vi "5_VisualAD_HyperParam_Search.vi"() -> ()   [LabVIEW 2020]
uses:
  <vilib>/Ngene/DeepLTK Anomaly Detection Addon/Toolkit/API/Controls/NNPC_Coreset_Params.ctl
  <vilib>/Ngene/DeepLTK Anomaly Detection Addon/Toolkit/API/Controls/NNPC_Setup.ctl
  <vilib>/Ngene/Deep Learning Toolkit/Toolkit/NN_Data/API/NN_Dims(C,H,W).ctl
  <vilib>/Ngene/Deep Learning Toolkit/Toolkit/NN_Network/Controls/NN_Device.ctl
  <vilib>/Ngene/DeepLTK Anomaly Detection Addon/Toolkit/API/Controls/Feature_Scorer_Params.ctl
  <vilib>/Ngene/DeepLTK Anomaly Detection Addon/Toolkit/API/Controls/Gaussian_Blur.ctl
  <vilib>/Ngene/DeepLTK Anomaly Detection Addon/Toolkit/API/Controls/Evaluation_Metrics.ctl
  <vilib>/Ngene/DeepLTK Anomaly Detection Addon/Toolkit/API/Controls/Eval_Results.ctl
  <vilib>/Ngene/DeepLTK Anomaly Detection Addon/Toolkit/API/Controls/MinMax.ctl
  <vilib>/Ngene/DeepLTK Anomaly Detection Addon/Toolkit/API/Controls/NNPC_Random_Projection_CFG.ctl
  <vilib>/Ngene/DeepLTK Anomaly Detection Addon/Toolkit/API/Controls/Dim_Reduction_Method.ctl
  <vilib>/Ngene/DeepLTK Anomaly Detection Addon/Toolkit/API/Controls/NNFE_CFG.ctl
  <vilib>/Ngene/DeepLTK Anomaly Detection Addon/Toolkit/API/Controls/Layer_Selector.ctl
  <vilib>/Ngene/DeepLTK Anomaly Detection Addon/Toolkit/API/Controls/Feature_Layer_Selector.ctl
  <vilib>/Ngene/DeepLTK Anomaly Detection Addon/Toolkit/API/Controls/Interpolation_Selector.ctl
  subVIs/Dataset_Reader/Controls/Read_Options.ctl
  <vilib>/Ngene/DeepLTK Anomaly Detection Addon/Toolkit/API/Controls/NNPC_PreProcessing_Options.ctl
  <vilib>/Ngene/DeepLTK Anomaly Detection Addon/Toolkit/API/Controls/NNPC_DS_Stats.ctl
  <vilib>/Ngene/DeepLTK Anomaly Detection Addon/Toolkit/API/Controls/Image_Stats_RGB.ctl
  subVIs/HyperParam_Search/Controls/Model_Info_and_Report.ctl
  subVIs/HyperParam_Search/Controls/Feature_Layers_CFG.ctl
  <vilib>/Ngene/DeepLTK Anomaly Detection Addon/Toolkit/API/Controls/Eval_Config.ctl
  <vilib>/Ngene/DeepLTK Anomaly Detection Addon/Toolkit/API/NNPC_Generate_Embedding/NNPC_Generate_Embedding(Dataset).vi
  <vilib>/Ngene/DeepLTK Anomaly Detection Addon/Toolkit/API/NNPC_Predict/NNPC_Predict(Dataset).vi
  <vilib>/Ngene/Deep Learning Toolkit/Toolkit/NN_Data/subVIs/Dataset_Destroy/NN_Dataset_Destroy(In3D_Out3D).vi
  <vilib>/Ngene/DeepLTK Anomaly Detection Addon/Toolkit/DeepLTK_Anomaly_Detection_Addon.lvlib
  <vilib>/Ngene/Deep Learning Toolkit/Toolkit/Deep_Learning_Toolkit_by_Ngene.lvlib
panel:
  in  "Tab Control":enum32{"Setup", "Results"}(tab)
  in  "Min_Layers_In_Group":u16=1
  in  "Dataset_Path(Train/Test/GT)":path=path "D:/Ngene/GitHub/deepltk_examples/3_Image_Processing/36_Anomaly_Detection/Dataset/Playing_Cards_3ofHearts"
  in  "Destination_Path":path=path "D:/working"
  in  "Coreset_Size":i32[](array[numeric])=[1000, 2000, 5000, 10000]
  in  "Proj._Dim.":i32[](array[numeric])=[128, 256, 512]
  in  "Coreset_Params":T1={"CoreSet_Size"=1.0, "Start_idx"=3}
  in  "NNPC_Setup":T2={"Input_Dims"={"C"=3, "H"=224, "W"=224}, "mBatch"=1, "Device"=enum."GPU", "GPU Id"=0}
  in  "Feature_Scorer_Params":T5={"Nearest_Neighbors"=1, "Calculate Anomaly Map"=FALSE, "Gaussian_Blur"={"Kernel_Size"=33, "Sigma"=4.0}}
  in  "Dim Reduction":T7={"Method"=enum."Rnd_Proj", "Target_Dim"=-1, "Seed"=42}
  in  "NNFE_CFG":T9={"Name"="", "Layer_Selection_By"=enum."Stride", "Feature_Layers"={"[LayerID, PatchSize]"=[{"Layer_ID"=8, "Patch_Size"=3}, {"Layer_ID"=16, "Patch_Size"=3}]}, "Interpolation_Type"=enum."Bi-Linear"}
  in  "NNFE_Folder_Paths":path[](array[path])=[path "D:/Ngene/GitHub/deepltk_examples/3_Image_Processing/36_Anomaly_Detection/NNFE/WRN_50_2_2_L3"]
  in  "Patch Sizes":i32[](array[numeric])=[1, 3, 5]
  in  "Layer ID":i32[](array[numeric])=[8, 16]
  out "Generated_Feature_Layers":T11[](array[typedef])=[{"[LayerID, PatchSize]"=[{"Layer_ID"=16, "Patch_Size"=1}]}, {"[LayerID, PatchSize]"=[{"Layer_ID"=16, "Patch_Size"=3}]}, {"[LayerID, PatchSize]"=[{"Layer_ID"=16, "Patch_Size"=5}]}, {"[LayerID, PatchSize]"=[{"Layer_ID"=8, "Patch_Size"=1}]}, {"[LayerID, PatchSize]"=[{"Layer_ID"=8, "Patch_Size"=1}, {"Layer_ID"=16, "Patch_Size"=1}]}, {"[LayerID, PatchSize]"=[{"Layer_ID"=8, "Patch_Size"=1}, {"Layer_ID"=16, "Patch_Size"=3}]}, {"[LayerID, PatchSize]"=[{"Layer_ID"=8, "Patch_Size"=1}, {"Layer_ID"=16, "Patch_Size"=5}]}, {"[LayerID, PatchSize]"=[{"Layer_ID"=8, "Patch_Size"=3}]}, {"[LayerID, PatchSize]"=[{"Layer_ID"=8, "Patch_Size"=3}, {"Layer_ID"=16, "Patch_Size"=1}]}, {"[LayerID, PatchSize]"=[{"Layer_ID"=8, "Patch_Size"=3}, {"Layer_ID"=16, "Patch_Size"=3}]}, {"[LayerID, PatchSize]"=[{"Layer_ID"=8, "Patch_Size"=3}, {"Layer_ID"=16, "Patch_Size"=5}]}, {"[LayerID, PatchSize]"=[{"Layer_ID"=8, "Patch_Size"=5}]}, {"[LayerID, PatchSize]"=[{"Layer_ID"=8, "Patch_Size"=5}, {"Layer_ID"=16, "Patch_Size"=1}]}, {"[LayerID, PatchSize]"=[{"Layer_ID"=8, "Patch_Size"=5}, {"Layer_ID"=16, "Patch_Size"=3}]}, {"[LayerID, PatchSize]"=[{"Layer_ID"=8, "Patch_Size"=5}, {"Layer_ID"=16, "Patch_Size"=5}]}]
  in  "Max_Layers_In_Group":u16=2
  out "error out":errorcluster
  in  "Img Res. H":i32[](array[numeric])=[224, 256]
  in  "Img Res. W":i32[](array[numeric])=[224, 256]
  in  "Single DS?":bool=TRUE
  out "Img._W":i32=224
  out "Elapsed Time":dbl=122.46820600000501 format="%<%H:%M:%S>t"
  out "Max_Dist":sgl[](graph)
  out "Tot Itr of one DS":i32=360
  out "Current Iter":i32=72
  out "Coreset Size":i32=4
  out "Proj. Dim.":i32=3
  out "Img Res.":i32=2
  out "Feature_Layers":i32=15
  out "Elapsed Time":dbl=122.46820600000501
  out "Evaluation_Metrics(Image)":T13={"Scores(Good)"={"X Values"=[48.00461868286133, 48.32544052124023, 48.64626235961914, 48.96708419799805, 49.28790603637695, 49.60872787475586, 49.92954971313476, 50.25037155151367, 50.57119338989258, 50.89201522827148, 51.212837066650394, 51.5336589050293, 51.8544807434082, 52.17530258178711, 52.49612442016601, 52.816946258544924, 53.13776809692383, 53.45858993530273, 53.779411773681645, 54.10023361206055, 54.421055450439454, 54.74187728881836, 55.06269912719726, 55.383520965576174, 55.70434280395508, 56.02516464233398, 56.34598648071289, 56.6668083190918, 56.987630157470704, 57.30845199584961, 57.62927383422851, 57.950095672607425, 58.27091751098633, 58.591739349365234, 58.91256118774414, 59.23338302612305, 59.554204864501955, 59.87502670288086, 60.195848541259764, 60.516670379638676, 60.83749221801758, 61.158314056396485, 61.47913589477539, 61.7999577331543, 62.120779571533205, 62.44160140991211, 62.762423248291014, 63.083245086669926, 63.40406692504883, 63.724888763427735, 64.04571060180663, 64.36653244018555, 64.68735427856446, 65.00817611694336, 65.32899795532227, 65.64981979370117, 65.97064163208009, 66.29146347045898, 66.6122853088379, 66.93310714721679, 67.2539289855957, 67.57475082397461, 67.89557266235352, 68.21639450073243, 68.53721633911132, 68.85803817749024, 69.17886001586913, 69.49968185424805, 69.82050369262694, 70.14132553100586, 70.46214736938477, 70.78296920776367, 71.10379104614259, 71.42461288452148, 71.7454347229004, 72.06625656127929, 72.38707839965821, 72.70790023803711, 73.02872207641602, 73.34954391479492, 73.67036575317383, 73.99118759155274, 74.31200942993163, 74.63283126831055, 74.95365310668944, 75.27447494506836, 75.59529678344727, 75.91611862182617, 76.23694046020509, 76.55776229858398, 76.8785841369629, 77.19940597534179, 77.52022781372071, 77.84104965209961, 78.16187149047852, 78.48269332885742, 78.80351516723633, 79.12433700561525, 79.44515884399414, 79.76598068237305], "Histogram: h(x)"=[1, 0, 0, 0, 0, 0, 1, 0, 0, 0, 1, 0, 1, 0, 1, 0, 2, 2, 0, 0, 1, 2, 1, 0, 0, 0, 1, 1, 0, 1, 0, 0, 0, 0, 1, 0, 0, 0, 1, 0, 0, 1, 0, 0, 1, 0, 0, 0, 0, 0, 0, 0, 0, 0, 0, 1, 0, 0, 0, 0, 0, 0, 0, 0, 0, 0, 0, 1, 0, 1, 1, 0, 0, 0, 0, 0, 0, 0, 0, 0, 0, 1, 0, 0, 0, 0, 0, 0, 0, 0, 0, 0, 0, 0, 0, 0, 0, 0, 0, 0]}, "Scores(Bad)"={"X Values"=[48.00461868286133, 48.32544052124023, 48.64626235961914, 48.96708419799805, 49.28790603637695, 49.60872787475586, 49.92954971313476, 50.25037155151367, 50.57119338989258, 50.89201522827148, 51.212837066650394, 51.5336589050293, 51.8544807434082, 52.17530258178711, 52.49612442016601, 52.816946258544924, 53.13776809692383, 53.45858993530273, 53.779411773681645, 54.10023361206055, 54.421055450439454, 54.74187728881836, 55.06269912719726, 55.383520965576174, 55.70434280395508, 56.02516464233398, 56.34598648071289, 56.6668083190918, 56.987630157470704, 57.30845199584961, 57.62927383422851, 57.950095672607425, 58.27091751098633, 58.591739349365234, 58.91256118774414, 59.23338302612305, 59.554204864501955, 59.87502670288086, 60.195848541259764, 60.516670379638676, 60.83749221801758, 61.158314056396485, 61.47913589477539, 61.7999577331543, 62.120779571533205, 62.44160140991211, 62.762423248291014, 63.083245086669926, 63.40406692504883, 63.724888763427735, 64.04571060180663, 64.36653244018555, 64.68735427856446, 65.00817611694336, 65.32899795532227, 65.64981979370117, 65.97064163208009, 66.29146347045898, 66.6122853088379, 66.93310714721679, 67.2539289855957, 67.57475082397461, 67.89557266235352, 68.21639450073243, 68.53721633911132, 68.85803817749024, 69.17886001586913, 69.49968185424805, 69.82050369262694, 70.14132553100586, 70.46214736938477, 70.78296920776367, 71.10379104614259, 71.42461288452148, 71.7454347229004, 72.06625656127929, 72.38707839965821, 72.70790023803711, 73.02872207641602, 73.34954391479492, 73.67036575317383, 73.99118759155274, 74.31200942993163, 74.63283126831055, 74.95365310668944, 75.27447494506836, 75.59529678344727, 75.91611862182617, 76.23694046020509, 76.55776229858398, 76.8785841369629, 77.19940597534179, 77.52022781372071, 77.84104965209961, 78.16187149047852, 78.48269332885742, 78.80351516723633, 79.12433700561525, 79.44515884399414, 79.76598068237305], "Histogram: h(x)"=[0, 0, 0, 0, 0, 0, 0, 0, 0, 0, 0, 0, 0, 0, 0, 0, 0, 0, 0, 0, 0, 0, 0, 0, 0, 0, 0, 0, 0, 0, 0, 0, 0, 0, 0, 0, 0, 0, 0, 0, 0, 0, 0, 0, 0, 0, 0, 0, 0, 0, 0, 0, 0, 0, 0, 0, 0, 0, 1, 0, 0, 0, 0, 0, 0, 1, 0, 0, 1, 3, 0, 1, 0, 1, 2, 0, 1, 0, 3, 2, 1, 1, 0, 2, 0, 1, 1, 0, 0, 1, 0, 0, 0, 0, 1, 0, 0, 0, 0, 1]}, "Eval Stats"={"Scores(Good)"={"Min"=47.844208, "Max"=73.85858}, "Scores(Bad)"={"Min"=66.62182, "Max"=79.92639}, "# of Samples(Good)"=25, "# of Samples(Bad)"=25, "AUROC"=0.9544, "F1_Max"=0.92592597, "Thrshld(F1_Max)"=65.82822, "Prec.(F1_Max)"=0.86206895, "Recall(F1_Max)"=1.0, "FPR(F1_Max)"=0.16, "FNR(F1_Max)"=0.0}} {"Eval Stats"."Recall(F1_Max)" format="%#.5f"; "Eval Stats"."FPR(F1_Max)" format="%#.5f"; "Eval Stats"."FNR(F1_Max)" format="%#.5f"; "Eval Stats"."Prec.(F1_Max)" format="%#.5f"; "Eval Stats"."F1_Max" format="%#.5f"; "Eval Stats"."AUROC" format="%#.5f"; "Eval Stats"."Scores(Bad)"."Min" format="%#_5g"; "Eval Stats"."Scores(Good)"."Min" format="%#_5g"; "Eval Stats"."Thrshld(F1_Max)" format="%#_5f"}
  out "Evaluation_Metrics(Pixel)":T13 {"Eval Stats"."Recall(F1_Max)" format="%#.5f"; "Eval Stats"."FPR(F1_Max)" format="%#.5f"; "Eval Stats"."FNR(F1_Max)" format="%#.5f"; "Eval Stats"."Prec.(F1_Max)" format="%#.5f"; "Eval Stats"."F1_Max" format="%#.5f"; "Eval Stats"."AUROC" format="%#.5f"; "Eval Stats"."Scores(Bad)"."Min" format="%#_5g"; "Eval Stats"."Scores(Good)"."Min" format="%#_5g"; "Eval Stats"."Thrshld(F1_Max)" format="%#_5f"}
  out "Coreset Size":i32
  out "Coreset Size":i32=10000
  out "Proj. Dim.":i32=128
  out "Img._H":i32=224
  out "Proj. Dim.":i32
  out "Img Res.":i32
  out "dT_Eval":dbl=0.0058932999963872135 format="%#_4p"
  out "dT_Inference":dbl=0.00638807999988785 format="%#_4p"
  out "dT_Coreset":dbl=3.193082099998719 format="%#_4p"
  out "dT_Embed":dbl=0.3958723999967333 format="%#_3p"
  out "dT_Init":dbl=1.9861645999917528 format="%#_3p"
  out "dT_DS_Read(Test)":dbl=0.14525060000596568 format="%#_3p"
  out "dT_DS_Read(Train)":dbl=0.18623009999282658 format="%#_3p"
  out "DS Size(Test)":i32=50
  out "DS Size(Train)":i32=50
  out "Feature_Layers":i32=6
  out "dT_DS_Read(Train)":dbl=0.18623009999282658 format="%#.0f"
  out "dT_DS_Read(Test)":dbl=0.14525060000596568 format="%#.0f"
  out "dT_Init":dbl=34.90064259998326 format="%#.0f"
  out "dT_Predict":dbl=21.941430500039132 format="%#.0f"
  out "dT_Coreset":dbl=53.35089359995618 format="%#.0f"
  out "dT_Embed":dbl=7.164398699984304 format="%#.0f"
  out "dT_Eval":dbl=0.4300707999354927 format="%#.0f"
  out "Feature Extractor":string="wrn_50_2_2_bnmerge"
  out "dT_Predict":dbl=0.3194039999943925
  out "[LayerID, PatchSize]":cluster{"Layer_ID":i32, "Patch_Size":i32}[](array[cluster])=[{"Layer_ID"=8, "Patch_Size"=1}, {"Layer_ID"=16, "Patch_Size"=5}]
  in  "Stop":bool
  out "NNFE":i32
  out "NNFE":i32=1
  out "Best_Model":string="16_wrn_50_2_2_bnmerge_Res224x224_L16P3_Prj256_CSet10k"
  out "Best_AUC":sgl=1.0 format="%#_5g"
  out "DS":i32=1
  out "DS":i32
  out "DS_Name":string="Playing_Cards_3ofHearts"
  out "Crrnt Iter":i32=72
  out "Total Iters":i32=360
  # "Total Iterations"
  # "Current Iteration"
  # "Current Settings"
  # "Total Times"
  # "Best Settings"
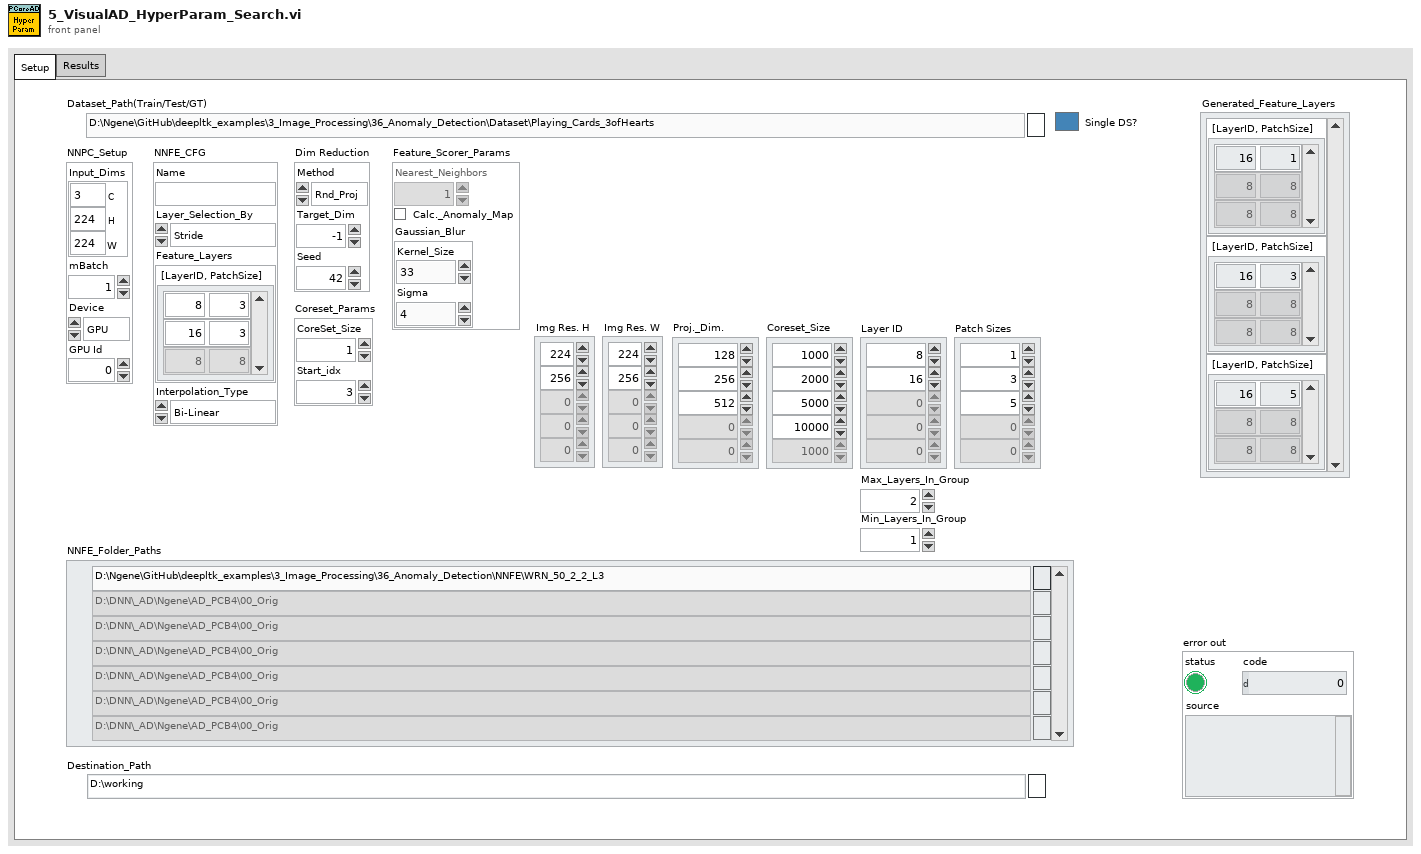
[diagram p1: front panel]
types:
  T1 = typedef "DeepLTK_Anomaly_Detection_Addon.lvlib/NNPC_Coreset_Params.ctl" = cluster{"CoreSet_Size":sgl, "Start_idx":i32}
  T2 = typedef "DeepLTK_Anomaly_Detection_Addon.lvlib/NNPC_Setup.ctl" = cluster{"Input_Dims":T3, "mBatch":i32, "Device":T4, "GPU Id":i32}
  T3 = typedef "Deep_Learning_Toolkit_by_Ngene.lvlib/NN_Dims(C,H,W).ctl" = cluster{"C":i32, "H":i32, "W":i32}
  T4 = typedef "Deep_Learning_Toolkit_by_Ngene.lvlib/NN_Device.ctl" = enum16{"CPU", "GPU"}
  T5 = typedef "DeepLTK_Anomaly_Detection_Addon.lvlib/Feature_Scorer_Params.ctl" = cluster{"Nearest_Neighbors":i32, "Calculate Anomaly Map":bool, "Gaussian_Blur":T6}
  T6 = typedef "DeepLTK_Anomaly_Detection_Addon.lvlib/Gaussian_Blur.ctl" = cluster{"Kernel_Size":i32, "Sigma":sgl}
  T7 = typedef "DeepLTK_Anomaly_Detection_Addon.lvlib/NNPC_Random_Projection_CFG.ctl" = cluster{"Method":T8, "Target_Dim":i32, "Seed":i32}
  T8 = typedef "DeepLTK_Anomaly_Detection_Addon.lvlib/Dim_Reduction_Method.ctl" = enum16{"None", "Rnd_Proj", "PCA"}
  T9 = typedef "DeepLTK_Anomaly_Detection_Addon.lvlib/NNFE_CFG.ctl" = cluster{"Name":string, "Layer_Selection_By":T10, "Feature_Layers":T11, "Interpolation_Type":T12}
  T10 = typedef "DeepLTK_Anomaly_Detection_Addon.lvlib/Layer_Selector.ctl" = enum16{"Stride", "Layer_Idx"}
  T11 = typedef "DeepLTK_Anomaly_Detection_Addon.lvlib/Feature_Layer_Selector.ctl" = cluster{"[LayerID, PatchSize]":cluster{"Layer_ID":i32, "Patch_Size":i32}[]}
  T12 = typedef "DeepLTK_Anomaly_Detection_Addon.lvlib/Interpolation_Selector.ctl" = enum16{"Nearest", "Bi-Linear"}
  T13 = typedef "DeepLTK_Anomaly_Detection_Addon.lvlib/Evaluation_Metrics.ctl" = cluster{"Scores(Good)":cluster{"X Values":dbl[], "Histogram: h(x)":i32[]}, "Scores(Bad)":cluster{"X Values":dbl[], "Histogram: h(x)":i32[]}, "Eval Stats":T14}
  T14 = typedef "DeepLTK_Anomaly_Detection_Addon.lvlib/Eval_Results.ctl" = cluster{"Scores(Good)":T15, "Scores(Bad)":T15, "# of Samples(Good)":i32, "# of Samples(Bad)":i32, "AUROC":sgl, "F1_Max":sgl, "Thrshld(F1_Max)":sgl, "Prec.(F1_Max)":sgl, "Recall(F1_Max)":sgl, "FPR(F1_Max)":sgl, "FNR(F1_Max)":sgl}
  T15 = typedef "DeepLTK_Anomaly_Detection_Addon.lvlib/MinMax.ctl" = cluster{"Min":sgl, "Max":sgl}
  T16 = typedef "DeepLTK_Anomaly_Detection_Addon.lvlib/NN_Paths.ctl" = cluster{"CFG":path, "BIN":path}
  T17 = enum16{"open", "replace", "create", "open or create", "replace or create", "replace or create with confirmation"}
  T18 = typedef "DeepLTK_Anomaly_Detection_Addon.lvlib/NNPC_PreProcessing_Options.ctl" = cluster{"DS_Name":string, "Input_Dims":T3, "Center Crop Size":i32, "Interpolation Type":u32, "Multi-Stage_DownSample?":bool, "Dataset_Stats":T19}
  T19 = typedef "DeepLTK_Anomaly_Detection_Addon.lvlib/NNPC_DS_Stats.ctl" = cluster{"means":T20, "stds":T20}
  T20 = typedef "DeepLTK_Anomaly_Detection_Addon.lvlib/Image_Stats_RGB.ctl" = cluster{"R":sgl, "G":sgl, "B":sgl}
  T21 = typedef "Read_Options.ctl" = cluster{"Read Bads?":bool, "Read GTs?":bool, "Update. DS Stats?":bool}
  T22 = typedef "DeepLTK_Anomaly_Detection_Addon.lvlib/Eval_Config.ctl" = cluster{"Extract_Good_Pixels_from_Bad":bool, "# bins":i32}
  T23 = typedef "Model_Info_and_Report.ctl" = cluster{"Name":string, "Feature Extractor":string, "Input3D_Custom_Dims":T3, "Coreset Size":i32, "J-L Proj. Dim.":i32, "Train_Time":dbl, "Inf_Time":dbl, "Feature_Layers":T24, "Eval Stats(Image)":T14, "Eval Stats(Pixel)":T14}
  T24 = typedef "Feature_Layers_CFG.ctl" = cluster{"Layer_ID":i32, "Patch_Size":i32}[]
  T25 = typedef "Deep_Learning_Toolkit_by_Ngene.lvlib/NN_DataSet(In3D_Out3D).ctl" = cluster{"Dataset_Size":i32, "Dims_In":T3, "Labels":string[], "File Paths":path[], "Outputs Ref.":T26, "Inputs Ref.":variant, "Dims_Out":T3}
  T26 = typedef "Deep_Learning_Toolkit_by_Ngene.lvlib/NN_Data_ref(4D_SGL).ctl" = refnum<data-value>
  T27 = typedef "DeepLTK_Anomaly_Detection_Addon.lvlib/NNPC_Instance.ctl" = cluster{"NN out":T28, "MemBank_Data":T43, "Name":string}
  T28 = typedef "Deep_Learning_Toolkit_by_Ngene.lvlib/NN.ctl" = cluster{"Name":string, "No of Layers":i32, "mBatch":i32, "Layers":T29[], "Dimty":T30, "Dims_In":T3, "Dims_Out":T3, "Working_Dir":path, "Train?":bool, "Train_Params":T31, "LR_Update_Policy":T34, "Session Data":T36, "Ground_truth":T37, "NNg_hdls":T38, "NN_Device":T4, "GPU Id":i32, "Labels":string[], "Receptive Field":T39[], "Loss_Type":T40, "Loss_Cfg_Prms":variant, "NNG_WS":T41}
  T29 = typedef "Deep_Learning_Toolkit_by_Ngene.lvlib/NN_Layer_ref.ctl" = refnum<data-value>
  T30 = typedef "Deep_Learning_Toolkit_by_Ngene.lvlib/NN_In_Out_Dim-ty.ctl" = enum8{"In1D_Out1D", "In3D_Out1D", "In3D_Out3D", "In3D_OutBBox"}
  T31 = typedef "Deep_Learning_Toolkit_by_Ngene.lvlib/NN_Train_Params.ctl" = cluster{"Optimizer":T32, "Beta_1":sgl, "Beta_2":sgl, "Weight Decay(L1)":sgl, "Weight Decay(L2)":sgl, "Data_Sampling":T33}
  T32 = typedef "Deep_Learning_Toolkit_by_Ngene.lvlib/NN_Train_Optimizer.ctl" = enum16{"SGD", "Adam", "Adagrad", "Adadelta", "RMSProp", "Nesterov"}
  T33 = typedef "Deep_Learning_Toolkit_by_Ngene.lvlib/NN_Train_Data_Sampling.ctl" = enum16{"Random", "Sequential"}
  T34 = typedef "Deep_Learning_Toolkit_by_Ngene.lvlib/NN_LR_Policy_Cfg.ctl" = cluster{"Policy_Type":T35, "LR0":dbl, "k":sgl, "WarmUp_Policy":enum16{"Step", "Ramp"}, "WarmUp_Iter":i32, "WarmUp_Ratio":sgl}
  T35 = typedef "Deep_Learning_Toolkit_by_Ngene.lvlib/NN_LR_Policy_Type.ctl" = enum16{"Manual", "Step", "Exp", "1/t"}
  T36 = typedef "Deep_Learning_Toolkit_by_Ngene.lvlib/NN_Train_Session_Data.ctl" = cluster{"Epochs":sgl, "Tot_Iter":i32, "LR":sgl, "LR_iter":i32}
  T37 = typedef "Deep_Learning_Toolkit_by_Ngene.lvlib/NN_Ground_truth.ctl" = cluster{"Y":variant}
  T38 = typedef "Deep_Learning_Toolkit_by_Ngene.lvlib/nng_cuda_handles.ctl" = cluster{"cudnn":u64, "cublas":u64, "stream":u64, "curand":u64}
  T39 = typedef "Deep_Learning_Toolkit_by_Ngene.lvlib/NN_Dims(V,H).ctl" = cluster{"V":i32, "H":i32}
  T40 = typedef "Deep_Learning_Toolkit_by_Ngene.lvlib/NN_Loss_Type.ctl" = enum16{"None", "MSE", "CrossEntropy", "YOLO_v2", "YOLO_v4"}
  T41 = typedef "Deep_Learning_Toolkit_by_Ngene.lvlib/NNG_WS.ctl" = cluster{"NNG_WS_Mem":T42, "Max_WS_Size":i64}
  T42 = typedef "Deep_Learning_Toolkit_by_Ngene.lvlib/NNg_WS_Mem_DVR.ctl" = refnum<data-value>
  T43 = typedef "DeepLTK_Anomaly_Detection_Addon.lvlib/MemBank_and_Norm_Variants.ctl" = cluster{"MemBank":variant, "MemBank Norm":variant}
  T44 = typedef "DeepLTK_Anomaly_Detection_Addon.lvlib/Evaluation_Metrics(Pixel_Image).ctl" = cluster{"Evaluation_Metrics(Pixel)":T13, "Evaluation_Metrics(Image)":T13}
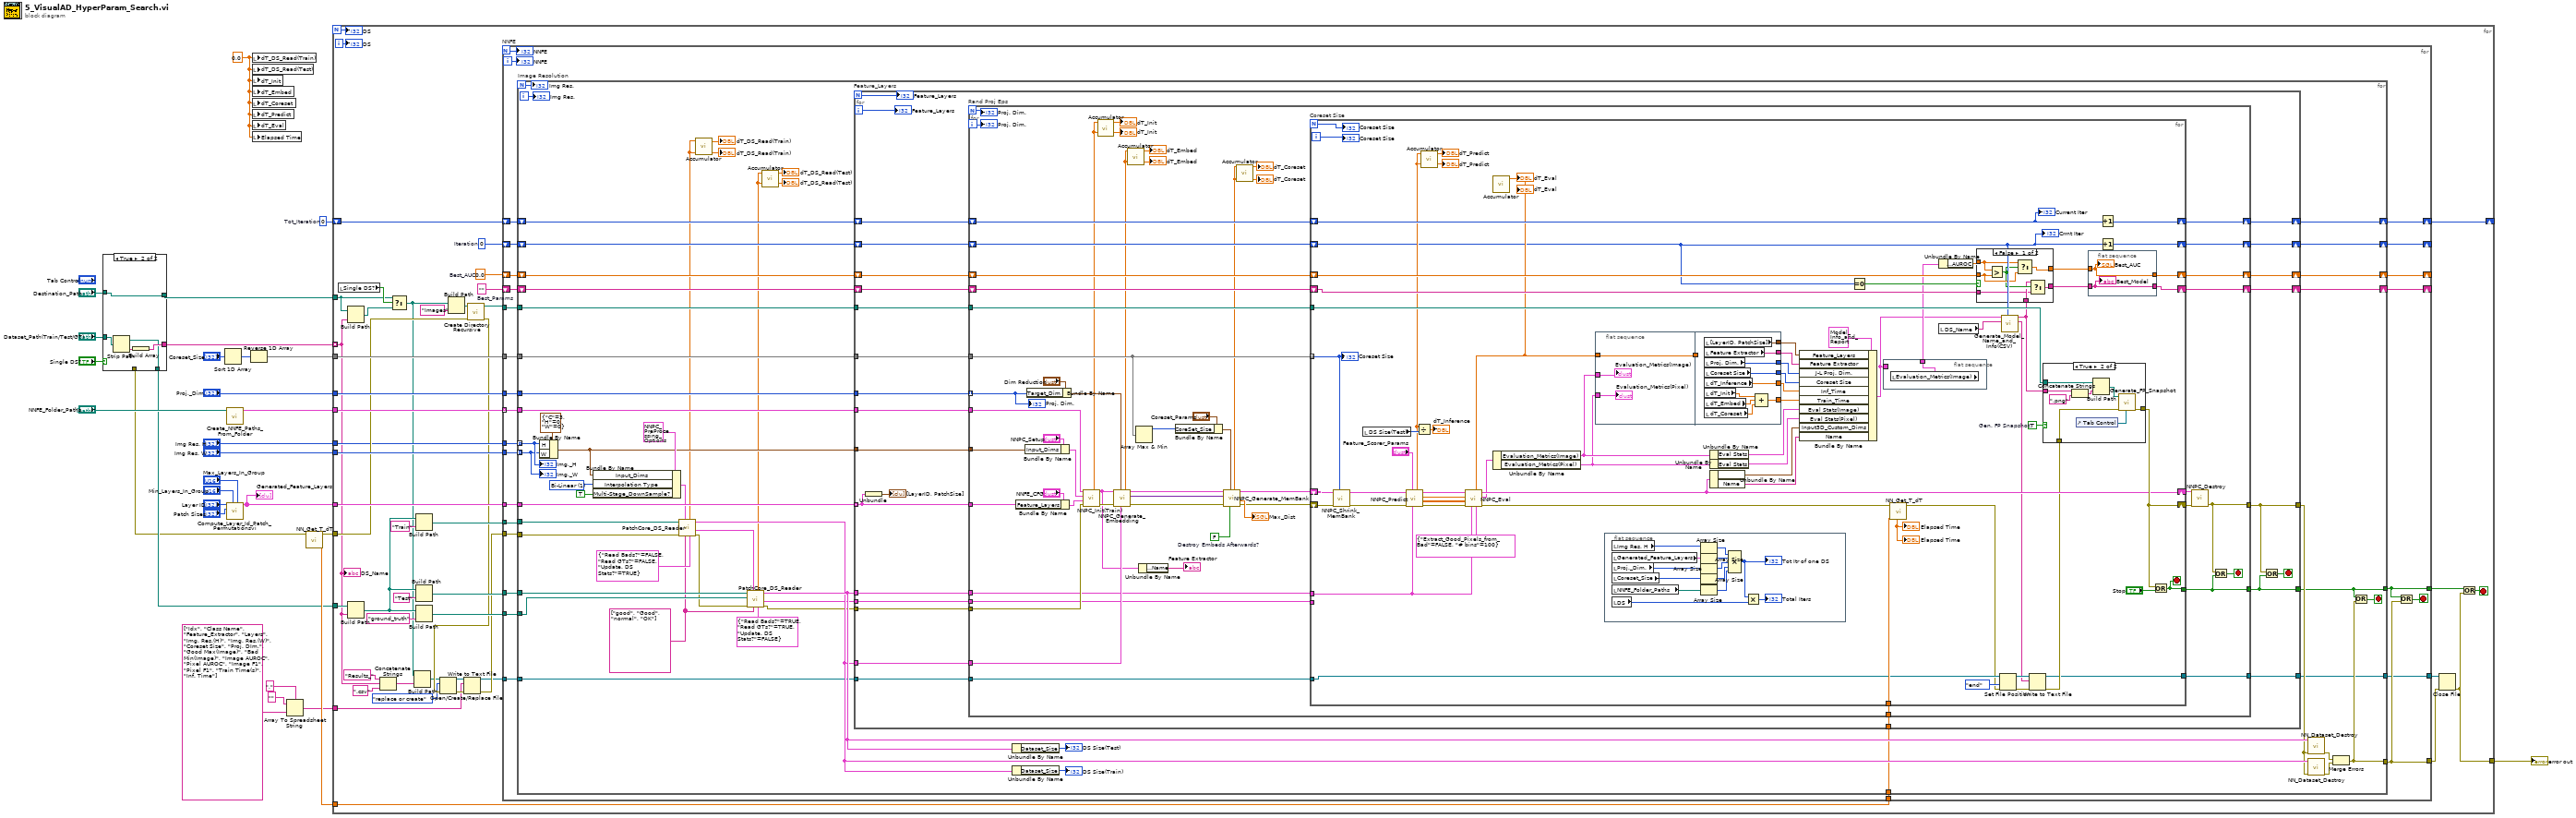
[diagram p0: block diagram]
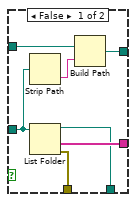
[diagram p4: hidden frame]
diagram:
  w5 = 0.0 ("dT_Eval")
  w17 = 0  # Tot_Iteration
  n1 = case shown="True" "Single DS?" {
    tunnel: "Dataset_Path(Train/Test/GT)" -> [w31 w39]
    tunnel: [w36 w40] -> w10
    tunnel: [w35 w38] -> w9
    tunnel: [w34 _] -> w8
    tunnel: "Destination_Path" -> [w32 w37]
    tunnel: [w30 w37] -> w6
    frame False {
      n2 = Strip Path(path=w31) -> (name=w33:string)  [unwired: 1 out]
      n3 = List Folder(path=w31) -> (path out=w35:path, folder names=w36:string[], error out=w34:errorcluster)  [unwired: 3 in, 1 out]
      n4 = Build Path(base path=w32, name or relative path=w33) -> (appended path=w30:path)
    }
    frame True {
      n5 = Strip Path(path=w39) -> (stripped path=w38:path, name=w41:string)
      n6 = Build Array(w41) -> (w40:string[])
    }
  }
  n7 = Sort 1D Array(array="Coreset_Size") -> (sorted array=w27:i32[])
  n8 = call "Create_NNFE_Paths_From_Folder.vi"("NNFE_Folder_Paths"="NNFE_Folder_Paths") -> ("NNFE_File_Paths"=w23:T16[])  [unwired: 10 in]
  n9 = call "Compute_Layer_Id_Patch_Permutationsvi.vi"("Max_#Layers_in_a_Group"="Max_Layers_In_Group", "Min_#Layers_in_a_Group"="Min_Layers_In_Group", "Patch_Sizes"="Patch Sizes", "Layer_IDs"="Layer ID") -> ("LayerID,PatchSize Permutations"=w20:T11[])  [unwired: 7 in]
  "Generated_Feature_Layers" <- w20
  n10 = Reverse 1D Array(array=w27) -> (reversed array=w26:i32[])
  n11 = local write "dT_DS_Read(Train)"(w5) -> ()
  n12 = local write "dT_DS_Read(Test)"(w5) -> ()
  n13 = local write "dT_Init"(w5) -> ()
  n14 = local write "dT_Embed"(w5) -> ()
  n15 = local write "dT_Coreset"(w5) -> ()
  n16 = local write "dT_Predict"(w5) -> ()
  n17 = local write "dT_Eval"(w5) -> ()
  n18 = local write "Elapsed Time"(w5) -> ()
  n19 = Array To Spreadsheet String(delimiter (Tab)=",", array=string[] ["Idx", "Class Name", "Feature_Extractor", "Layers", "Img. Res.(H)", "Img. Res.(W)", "Coreset Size", "Proj. DIm.", "Good Max(Image)", "Bad Min(Image)", "Image AUROC", "Pixel AUROC", "Image F1", "Pixel F1", "Train Time(s)", "Inf. Time"] ("spreadsheet string"), 3:"" ("spreadsheet string")) -> (spreadsheet string=w1:string)
  n20 = call <vilib>:"NN_Get_T_dT.vi"("error in"=w8) -> ("T_out"=w16:dbl, "error out"=w15:errorcluster)  [unwired: 6 in, 1 out]
  n21 = for {
    N -> [w68]
    tunnel: "Img Res. W" -> [w88]
    tunnel: "Proj._Dim." -> [w87]
    tunnel: w26 -> [w85]
    tunnel: w23 -> [w84]
    tunnel: w20 -> [w83]
    tunnel: w10 -> [w49] mode=indexing
    tunnel: w6 -> [w59]
    tunnel: w9 -> [w70]
    shift-right: [w66] -> _
    shift-left: w17 -> [w67]
    tunnel: w16 -> [w65]
    tunnel: "Img Res. H" -> [w63]
    tunnel: w15 -> [w71]
    tunnel: [w42] -> w24
    tunnel: w1 -> [w45]
    i -> [w64]
    stop <- w62 stop-if-true
    w81 = ""  # Best_Params
    w82 = sgl 0.0  # Best_AUC
    w86 = 0  # Iteration
    n22 = local read "Single DS?"() -> (w60:bool)
    n23 = Build Path(base path=w59, name or relative path=w49) -> (appended path=w58:path)
    n24 = Build Path(base path=w70, name or relative path=w49) -> (appended path=w69:path)
    n25 = Concatenate Strings("Results_" ("string"), w49, ".csv" ("string")) -> (w51:string)
    n26 = Select(t=w59, s=w60, f=w58) -> (s? t:f=w48:path)
    n27 = Build Path(base path=w48, name or relative path=w51) -> (appended path=w55:path)
    n28 = Build Path(base path=w69, name or relative path="Train" ("String")) -> (appended path=w77:path)
    n29 = Build Path(base path=w69, name or relative path="Test" ("String")) -> (appended path=w75:path)
    n30 = Build Path(base path=w69, name or relative path="ground_truth" ("String")) -> (appended path=w76:path)
    n31 = Build Path(base path=w48, name or relative path="Images" ("String")) -> (appended path=w74:path)
    n32 = call <vilib>:"Create Directory Recursive.vi"("error in (no error)"=w71, "directory"=w74) -> ("error out"=w57:errorcluster, "directory copy"=w72:path)  [unwired: 3 in, 1 out]
    n33 = Open/Create/Replace File(file path (use dialog)=w55, error in=w57, operation (0:open)=T17."replace or create") -> (refnum out=w54:refnum<file>, error out=w53:errorcluster)  [unwired: 3 in, 1 out]
    n34 = Write to Text File(file (use dialog)=w54, text=w45, error in=w53) -> (refnum out=w46:refnum<file>, error out=w47:errorcluster)  [unwired: 1 in, 1 out]
    n35 = for "NNFE" {
      N -> [w102]
      tunnel: w88 -> [w115]
      tunnel: w76 -> [w114]
      tunnel: w87 -> [w113]
      tunnel: w75 -> [w112]
      tunnel: w77 -> [w111]
      tunnel: w72 -> [w110]
      tunnel: w65 -> [w109]
      tunnel: w83 -> [w108]
      tunnel: w85 -> [w106]
      tunnel: w84 -> [w104] mode=indexing
      shift-right: [w103] -> _
      shift-left: w86 -> [w107]
      shift-right: [w100] -> _
      shift-left: w82 -> [w101]
      shift-right: [w98] -> _
      shift-left: w81 -> [w99]
      shift-right: [w96] -> w66
      shift-left: w67 -> [w97]
      tunnel: w63 -> [w94]
      tunnel: w47 -> [w105]
      tunnel: [w92] -> w43
      tunnel: [w91] -> w61
      tunnel: w46 -> [w90]
      tunnel: [w89] -> w44
      i -> [w95]
      stop <- w93 stop-if-true
      n36 = for "Image Resolution" {
        N -> [w143]
        tunnel: w114 -> [w162]
        tunnel: w111 -> [w163]
        tunnel: w115 -> [w120] mode=indexing
        tunnel: w113 -> [w166]
        tunnel: w106 -> [w165]
        tunnel: w112 -> [w161]
        tunnel: w110 -> [w153]
        tunnel: w109 -> [w152]
        tunnel: w108 -> [w144]
        shift-right: [w141] -> w103
        shift-left: w107 -> [w142]
        tunnel: w104 -> [w135]
        shift-right: [w132] -> w100
        shift-left: w101 -> [w133]
        shift-right: [w130] -> w98
        shift-left: w99 -> [w131]
        shift-right: [w128] -> w96
        shift-left: w97 -> [w129]
        tunnel: w94 -> [w121] mode=indexing
        tunnel: w105 -> [w164]
        tunnel: [w119] -> w92
        tunnel: [w118] -> w91
        tunnel: w90 -> [w117]
        tunnel: [w116] -> w89
        i -> [w126]
        stop <- w140 stop-if-true
        w150 = u32 1 items=["Zero Order", "Bi-Linear", "Quadratic", "Cubic Spline"] ("Interpolation Type")
        w136 = string[] ["good", "Good", "normal", "OK"] ("Good Folder Name")
        n37 = Bundle By Name(cluster=T3 {"C"=3, "H"=0, "W"=0} ("Input_Dims"), "H"=w121, "W"=w120) -> (w145:T3)
        n38 = Bundle By Name(cluster=T18 {"DS_Name"="", "Input_Dims"={"C"=4, "H"=224, "W"=224}, "Center Crop Size"=-1, "Interpolation Type"=1, "Multi-Stage_DownSample?"=FALSE, "Dataset_Stats"={"means"={"R"=0.5385, "G"=0.5348, "B"=0.551}, "stds"={"R"=0.3673, "G"=0.3673, "B"=0.3505}}} ("PreProcessing_Options"), "Input_Dims"=w145, "Interpolation Type"=w150, "Multi-Stage_DownSample?"=TRUE) -> (w138:T18)
        n39 = call "PatchCore_DS_Reader.vi"("Read Options"=T21 {"Read Bads?"=FALSE, "Read GTs?"=FALSE, "Update. DS Stats?"=TRUE}, "Good Unique Labels"=w136, "PreProc_Options_in"=w138, "error in (no error)"=w164, "Folder Path"=w163) -> ("error out"=w160:errorcluster, "PreProc_Options_out"=w137:T18, "Dataset"=w155:T25, "dT_DS_Reader"=w125:dbl)  [unwired: 3 in]
        "dT_DS_Read(Train)" <- w125
        n40 = call "Accumulator.vi"("in"=w125) -> ("accumulate_out"=→"dT_DS_Read(Train)":dbl)  [unwired: 10 in]
        n41 = call "PatchCore_DS_Reader.vi"("Read Options"=T21 {"Read Bads?"=TRUE, "Read GTs?"=TRUE, "Update. DS Stats?"=FALSE}, "Good Unique Labels"=w136, "PreProc_Options_in"=w137, "error in (no error)"=w160, "GT Folder Path"=w162, "Folder Path"=w161) -> ("error out"=w127:errorcluster, "PreProc_Options_out"=w147:T18, "Dataset"=w156:T25, "dT_DS_Reader"=w123:dbl)  [unwired: 2 in]
        "dT_DS_Read(Test)" <- w123
        n42 = call "Accumulator.vi"("in"=w123) -> ("accumulate_out"=→"dT_DS_Read(Test)":dbl)  [unwired: 10 in]
        n43 = for "Feature_Layers" {
          N -> [w183]
          tunnel: w166 -> [w193]
          tunnel: w165 -> [w192]
          tunnel: w156 -> [w190]
          tunnel: w155 -> [w189]
          tunnel: w153 -> [w188]
          tunnel: w152 -> [w187]
          tunnel: w147 -> [w186]
          tunnel: w145 -> [w185]
          tunnel: w144 -> [w184] mode=indexing
          tunnel: [w182] -> w118
          shift-right: [w181] -> w141
          shift-left: w142 -> [w180]
          tunnel: w135 -> [w176]
          shift-right: [w174] -> w132
          shift-left: w133 -> [w175]
          shift-right: [w172] -> w130
          shift-left: w131 -> [w173]
          shift-right: [w170] -> w128
          shift-left: w129 -> [w171]
          tunnel: w127 -> [w191]
          tunnel: [w178] -> w139
          tunnel: w117 -> [w168]
          tunnel: [w167] -> w116
          i -> [w169]
          stop <- w179 stop-if-true
          n44 = Unbundle(w184) -> ("[LayerID, PatchSize]"=→"[LayerID, PatchSize]":cluster{"Layer_ID":i32, "Patch_Size":i32}[])
          n45 = for "Rand Proj Eps" {
            N -> [w231]
            tunnel: w189 -> [w243]
            tunnel: w193 -> [w238] mode=indexing
            tunnel: w192 -> [w212]
            tunnel: w190 -> [w241]
            tunnel: w188 -> [w240]
            tunnel: w187 -> [w239]
            tunnel: w186 -> [w237]
            tunnel: w185 -> [w233]
            tunnel: w184 -> [w232]
            tunnel: [w230] -> w182
            shift-right: [w228] -> w181
            shift-left: w180 -> [w229]
            tunnel: w176 -> [w211]
            shift-right: [w208] -> w174
            shift-left: w175 -> [w209]
            shift-right: [w206] -> w172
            shift-left: w173 -> [w207]
            shift-right: [w204] -> w170
            shift-left: w171 -> [w205]
            tunnel: w191 -> [w246]
            tunnel: [w226] -> w178
            tunnel: w168 -> [w195]
            tunnel: [w194] -> w167
            i -> [w202]
            stop <- w227 stop-if-true
            w218 = FALSE  # Destroy Embeds Afterwards?
            n46 = Bundle By Name(cluster="NNFE_CFG", "Feature_Layers"=w232) -> (w225:T9)
            n47 = Bundle By Name(cluster="NNPC_Setup", "Input_Dims"=w233) -> (w224:T2)
            n48 = Bundle By Name(cluster="Dim Reduction", "Target_Dim"=w238) -> (w223:T7)
            n49 = call <vilib>:"NNPC_Init(Train).vi"("error in"=w246, "NNFE_CFG"=w225, "NNPC_Setup"=w224, "NNFE_Paths"=w211) -> ("error out"=w244:errorcluster, "NNPC_out"=w222:T27, "dT_Init_Train"=w198:dbl)  [unwired: 5 in]
            "dT_Init" <- w198
            n50 = call "Accumulator.vi"("in"=w198) -> ("accumulate_out"=→"dT_Init":dbl)  [unwired: 10 in]
            n51 = call-poly <vilib>:"NNPC_Generate_Embedding.vi"("Dataset"=w243, "Dim_Reduction"=w223, "error in"=w244, "NNPC_in"=w222) -> ("error out"=w217:errorcluster, "Feature_Embeddings"=w216:variant, "NNPC_out"=w215:T27, "dT_Embed"=w197:dbl)  [unwired: 3 in, 1 out]
            "dT_Embed" <- w197
            n52 = call "Accumulator.vi"("in"=w197) -> ("accumulate_out"=→"dT_Embed":dbl)  [unwired: 10 in]
            n53 = Array Max & Min(array=w212) -> (max value=w214:i32)  [unwired: 3 out]
            n54 = Unbundle By Name(w222) -> ("NN out.Name"=→"Feature Extractor":string)
            n55 = Bundle By Name(cluster="Coreset_Params", "CoreSet_Size"=w214) -> (w220:T1)
            n56 = call <vilib>:"NNPC_Generate_MemBank.vi"("Destroy Embeds Afterwards?"=w218, "Coreset_Params"=w220, "error in (no error)"=w217, "Feature_Embeddings"=w216, "NNPC_in"=w215) -> ("error out"=w203:errorcluster, "Max_Distances"=→"Max_Dist":sgl[], "NNPC_out"=w213:T27, "dT_Coreset"=w196:dbl)  [unwired: 3 in]
            "dT_Coreset" <- w196
            n57 = call "Accumulator.vi"("in"=w196) -> ("accumulate_out"=→"dT_Coreset":dbl)  [unwired: 10 in]
            n58 = for "Coreset Size" {
              N -> [w296]
              shift-right: [w264] -> w245
              shift-left: w213 -> [w290]
              shift-right: [w285] -> w242
              shift-left: w203 -> [w289]
              tunnel: w241 -> [w308]
              tunnel: w240 -> [w301]
              tunnel: w239 -> [w300]
              tunnel: w237 -> [_]
              tunnel: [w295] -> w230
              shift-right: [w280] -> w228
              shift-left: w229 -> [w260]
              tunnel: w212 -> [w288] mode=indexing
              shift-right: [w276] -> w208
              shift-left: w209 -> [w283]
              shift-right: [w277] -> w206
              shift-left: w207 -> [w282]
              shift-right: [w279] -> w204
              shift-left: w205 -> [w278]
              tunnel: w195 -> [w253]
              tunnel: [w249] -> w194
              i -> [w275]
              stop <- w295 stop-if-true
              w302 = TRUE  # Gen. FP Snapshot?
              n59 = call <vilib>:"NNPC_Shrink_MemBank.vi"("Coreset_Size"=w288, "error in (no error)"=w289, "NNPC_in"=w290) -> ("error out"=w265:errorcluster, "NNPC_out"=w266:T27)  [unwired: 7 in]
              n60 = local read "DS Size(Test)"() -> (w306:i32)
              n61 = call-poly <vilib>:"NNPC_Predict.vi"("Dataset"=w308, "Feature_Scorer_Params"="Feature_Scorer_Params", "error in (no error)"=w265, "NNPC_in"=w266) -> ("error out"=w311:errorcluster, "Anomaly_Maps"=w310:sgl[][][], "Pred_Scores"=w312:sgl[], "NNPC_out"=w313:T27, "dT_Predict"=w273:dbl)  [unwired: 3 in]
              "dT_Predict" <- w273
              n62 = Divide(x=w273, y=w306) -> (x/y=→"dT_Inference":dbl)
              n63 = call "Accumulator.vi"("in"=w273) -> ("accumulate_out"=→"dT_Predict":dbl)  [unwired: 10 in]
              n64 = call <vilib>:"NNPC_Eval.vi"("Eval_Config"=T22 {"Extract_Good_Pixels_from_Bad"=FALSE, "# bins"=100} ("Eval Config"), "Dataset"=w308, "error in (no error)"=w311, "Anomaly_Maps"=w310, "Pred_Scores"=w312, "NNPC_in"=w313) -> ("error out"=w263:errorcluster, "Evaluation_Metrics"=w262:T44, "NNPC_out"=w264:T27, "dT_Eval"=w271:dbl)  [unwired: 2 in]
              "dT_Eval" <- w271
              n65 = call "Accumulator.vi"("in"=w271) -> ("accumulate_out"=→"dT_Eval":dbl)  [unwired: 10 in]
              n66 = Unbundle By Name(w262) -> ("Evaluation_Metrics(Image)"=w293:T13, "Evaluation_Metrics(Pixel)"=w292:T13)
              n67 = flat-sequence {
                tunnel: w271 -> [w342]
                tunnel: [w342] -> w294
                tunnel: w292 -> [w341]
                tunnel: w293 -> [w340]
                tunnel: [w348] -> w305
                tunnel: [w347] -> w299
                tunnel: [w346] -> w298
                tunnel: [w345] -> w297
                tunnel: w294 -> [_]
                tunnel: [w344] -> w291
                tunnel: [w343] -> w287
                frame #0 {
                  "Evaluation_Metrics(Image)" <- w340
                  "Evaluation_Metrics(Pixel)" <- w341
                }
                frame #1 {
                  n68 = local read "[LayerID, PatchSize]"() -> (w343:cluster{"Layer_ID":i32, "Patch_Size":i32}[])
                  n69 = local read "Feature Extractor"() -> (w344:string)
                  n70 = local read "Proj. Dim."() -> (w345:i32)
                  n71 = local read "Coreset Size"() -> (w346:i32)
                  n72 = local read "dT_Inference"() -> (w347:dbl)
                  n73 = local read "dT_Init"() -> (w351:dbl)
                  n74 = local read "dT_Embed"() -> (w350:dbl)
                  n75 = local read "dT_Coreset"() -> (w349:dbl)
                  n76 = Compound Arithmetic op=ADD(w351, w350, w349) -> (w348:dbl)
                }
              }
              n77 = flat-sequence {
                frame #0 {
                  n78 = local read "Img Res. H"() -> (w327:i32[])
                  n79 = local read "Generated_Feature_Layers"() -> (w333:T11[])
                  n80 = local read "Proj._Dim."() -> (w339:i32[])
                  n81 = local read "Coreset_Size"() -> (w338:i32[])
                  n82 = local read "NNFE_Folder_Paths"() -> (w332:path[])
                  n83 = local read "DS"() -> (w328:i32)
                  n84 = Array Size(array=w327) -> (size(s)=w336:i32)
                  n85 = Array Size(array=w333) -> (size(s)=w337:i32)
                  n86 = Array Size(array=w339) -> (size(s)=w335:i32)
                  n87 = Array Size(array=w338) -> (size(s)=w334:i32)
                  n88 = Array Size(array=w332) -> (size(s)=w331:i32)
                  n89 = Compound Arithmetic op=MULTIPLY(w336, w337, w335, w334, w331) -> (w330:i32)
                  "Tot Itr of one DS" <- w330
                  n90 = Multiply(x=w330, y=w328) -> (x*y=→"Total Iters":i32)
                }
              }
              n91 = Unbundle By Name(w293) -> ("Eval Stats"=w304:T14)
              n92 = Unbundle By Name(w292) -> ("Eval Stats"=w303:T14)
              n93 = Unbundle By Name(w264) -> ("NN out.Dims_In"=w248:T3, "Name"=w247:string)
              n94 = Bundle By Name(cluster=T23 {"Name"="", "Feature Extractor"="wrn_50_2_2_bnmerge", "Input3D_Custom_Dims"={"C"=0, "H"=0, "W"=-1}, "Coreset Size"=0, "J-L Proj. Dim."=0, "Train_Time"=0.0, "Inf_Time"=0.0, "Feature_Layers"=[{"Layer_ID"=8, "Patch_Size"=3}, {"Layer_ID"=16, "Patch_Size"=3}], "Eval Stats(Image)"={"Scores(Good)"={"Min"=0.0, "Max"=0.0}, "Scores(Bad)"={"Min"=0.0, "Max"=0.0}, "# of Samples(Good)"=0, "# of Samples(Bad)"=0, "AUROC"=0.0, "F1_Max"=0.0, "Thrshld(F1_Max)"=0.0, "Prec.(F1_Max)"=0.0, "Recall(F1_Max)"=0.0, "FPR(F1_Max)"=0.0, "FNR(F1_Max)"=0.0}, "Eval Stats(Pixel)"={"Scores(Good)"={"Min"=0.0, "Max"=0.0}, "Scores(Bad)"={"Min"=0.0, "Max"=0.0}, "# of Samples(Good)"=0, "# of Samples(Bad)"=0, "AUROC"=0.0, "F1_Max"=0.0, "Thrshld(F1_Max)"=0.0, "Prec.(F1_Max)"=0.0, "Recall(F1_Max)"=0.0, "FPR(F1_Max)"=0.0, "FNR(F1_Max)"=0.0}} ("Model_Info_and_Report"), "Feature_Layers"=w287, "Feature Extractor"=w291, "J-L Proj. Dim."=w297, "Coreset Size"=w298, "Inf_Time"=w299, "Train_Time"=w305, "Eval Stats(Image)"=w304, "Eval Stats(Pixel)"=w303, "Input3D_Custom_Dims"=w248, "Name"=w247) -> (w259:T23)
              n95 = Equal To 0?(x=w260) -> (x = 0?=w270:bool)
              n96 = flat-sequence {
                tunnel: w259 -> [_]
                tunnel: [w315] -> w268
                frame #0 {
                  n97 = local read "Evaluation_Metrics(Image)"() -> (w315:T13)
                }
              }
              n98 = call <vilib>:"NN_Get_T_dT.vi"("T_in"=w300, "error in"=w263) -> ("error out"=w251:errorcluster, "dT"=→"Elapsed Time" →"Elapsed Time":dbl)  [unwired: 5 in, 1 out]
              n99 = Unbundle By Name(w268) -> ("Eval Stats.AUROC"=w267:sgl)
              n100 = local read "DS_Name"() -> (w258:string)
              n101 = Set File Position(refnum=w253, from (0:start)=enum16{"start", "end", "current"}."end", error in=w251) -> (refnum out=w256:refnum<file>, error out=w255:errorcluster)  [unwired: 1 in]
              n102 = call "Generate_Model_Name_and_Info(CSV).vi"("Iteration_idx"=w260, "DS_Name"=w258, "Model_Info_and_Report"=w259) -> ("Model_Info(CSV)"=w252:string, "Generated_Model_Name"=w257:string)  [unwired: 7 in]
              n103 = case shown="False" w270 {
                tunnel: [w322 w324] -> w284
                tunnel: w267 -> [w321 w324]
                tunnel: w283 -> [w320 _]
                tunnel: w257 -> [w318 w323]
                tunnel: w282 -> [w317 _]
                tunnel: [w316 w323] -> w281
                frame False {
                  n104 = Greater?(x=w321, y=w320) -> (0:w319:bool)
                  n105 = Select(t=w321, s=w319, f=w320) -> (s? t:f=w322:sgl)
                  n106 = Select(t=w318, s=w319, f=w317) -> (s? t:f=w316:string)
                }
                frame True {
                }
              }
              n107 = Write to Text File(file (use dialog)=w256, text=w252, error in=w255) -> (refnum out=w249:refnum<file>, error out=w250:errorcluster)  [unwired: 1 in, 1 out]
              n108 = case shown="True" w302 {
                tunnel: w301 -> [_ w356]
                tunnel: w250 -> [w352 w359]
                tunnel: [w352 w358] -> w285
                tunnel: w257 -> [_ w354]
                frame False {
                }
                frame True {
                  n109 = Concatenate Strings(w354, ".png" ("string")) -> (w353:string)
                  n110 = control-ref of="Tab Control"() -> (w360:refnum<vi>)
                  n111 = Build Path(base path=w356, name or relative path=w353) -> (appended path=w357:path)
                  n112 = call "Generate_FP_Snapshot.vi"("TabControl in"=w360, "error in"=w359, "File_Name"=w357) -> ("error out"=w358:errorcluster)  [unwired: 8 in]
                }
              }
              n113 = flat-sequence {
                tunnel: w284 -> [w326]
                tunnel: w281 -> [w325]
                tunnel: [w326] -> w276
                tunnel: [w325] -> w277
                frame #0 {
                  "Best_Model" <- w325
                  "Best_AUC" <- w326
                }
              }
              n114 = Increment(x=w278) -> (x+1=w279:i32)
              n115 = Increment(x=w260) -> (x+1=w280:i32)
              n116 = Or(x=w285, y="Stop") -> (x .or. y?=w295:bool)
              "Coreset Size" <- w275
              "Coreset Size" <- w296
              "Current Iter" <- w278
              "Coreset Size" <- w288
              "Crrnt Iter" <- w260
            }
            n117 = call <vilib>:"NNPC_Destroy.vi"("error in"=w242, "NNPC_in"=w245) -> ("error out"=w226:errorcluster)  [unwired: 9 in]
            n118 = Or(x=w226, y=w230) -> (x .or. y?=w227:bool)
            "Proj. Dim." <- w202
            "Proj. Dim." <- w238
            "Proj. Dim." <- w231
          }
          n119 = Or(x=w178, y=w182) -> (x .or. y?=w179:bool)
          "Feature_Layers" <- w169
          "Feature_Layers" <- w183
        }
        n120 = Unbundle By Name(w156) -> ("Dataset_Size"=→"DS Size(Test)":i32)
        n121 = Unbundle By Name(w155) -> ("Dataset_Size"=→"DS Size(Train)":i32)
        n122 = call-poly <vilib>:"NN_Dataset_Destroy.vi"("error in (no error)"=w139, "Dataset(In3D_Out3D)"=w156) -> ("error out"=w159:errorcluster)  [unwired: 9 in]
        n123 = call-poly <vilib>:"NN_Dataset_Destroy.vi"("error in (no error)"=w139, "Dataset(In3D_Out3D)"=w155) -> ("error out"=w154:errorcluster)  [unwired: 9 in]
        n124 = Merge Errors(w159, w154) -> (w119:errorcluster)
        n125 = Or(x=w118, y=w119) -> (x .or. y?=w140:bool)
        "Img Res." <- w126
        "Img._H" <- w121
        "Img Res." <- w143
        "Img._W" <- w120
      }
      n126 = Or(x=w91, y=w92) -> (x .or. y?=w93:bool)
      "NNFE" <- w102
      "NNFE" <- w95
    }
    n127 = Close File(refnum=w44, error in=w43) -> (error out=w42:errorcluster)  [unwired: 1 out]
    n128 = Or(x=w61, y=w42) -> (x .or. y?=w62:bool)
    "DS" <- w68
    "DS" <- w64
    "DS_Name" <- w49
  }
  "error out" <- w24
